vi "draw_quiver.vi"() -> ()   [LabVIEW 2016]
uses:
  <vilib>/Native 3D Graph/xcontrol/3DPC_SurfacePlot.xctl
  <vilib>/Native 3D Graph/classes/Line/Line.lvclass
panel:
  in  "XYZ Gain":dbl[](array[numeric])=[0.01, 0.01, 0.1]
  in  "XY Spacing":dbl=20.0 format="%#_13g"
  in  "Cols":i32=8
  in  "Rows":i32=8
  in  "Sensor Readings":dbl[][](array[numeric])=[[-533.0, -111.0, 239.0], [-402.0, 166.0, 184.0], [-184.0, 154.0, 29.0], [-106.0, 74.0, 11.0], [-532.0, -109.0, 246.0], [-398.0, 164.0, 175.0], [-205.0, 152.0, 32.0], [-119.0, 65.0, 9.0], [-529.0, -110.0, 242.0], [-408.0, 166.0, 184.0], [-198.0, 158.0, 27.0], [-108.0, 61.0, 6.0], [-539.0, -106.0, 240.0], [-407.0, 158.0, 183.0], [-191.0, 156.0, 28.0], [-113.0, 73.0, 15.0], [816.0, -260.0, 842.0], [539.0, 512.0, 512.0], [156.0, 425.0, 83.0], [13.0, 142.0, -72.0], [816.0, -262.0, 840.0], [528.0, 520.0, 512.0], [162.0, 425.0, 83.0], [13.0, 137.0, -84.0], [809.0, -260.0, 840.0], [538.0, 520.0, 504.0], [162.0, 432.0, 72.0], [13.0, 136.0, -84.0], [809.0, -260.0, 846.0], [538.0, 508.0, 512.0], [158.0, 435.0, 72.0], [19.0, 136.0, -79.0], [346.0, -168.0, 14.0], [287.0, -68.0, 19.0], [161.0, -34.0, 4.0], [70.0, -44.0, -7.0], [345.0, -191.0, 19.0], [279.0, -40.0, 8.0], [167.0, -16.0, 12.0], [72.0, -23.0, 2.0], [341.0, -190.0, 17.0], [285.0, -46.0, 9.0], [149.0, -15.0, 6.0], [54.0, -40.0, -2.0], [375.0, -201.0, 19.0], [282.0, -51.0, 10.0], [135.0, -37.0, 6.0], [81.0, -57.0, -12.0], [-80.0, -193.0, -48.0], [-73.0, -136.0, -12.0], [-5.0, -122.0, -31.0], [-19.0, -118.0, -17.0], [-118.0, -187.0, -48.0], [-73.0, -115.0, -22.0], [1.0, -113.0, -27.0], [-20.0, -111.0, -8.0], [-99.0, -184.0, -40.0], [-62.0, -145.0, -17.0], [0.0, -113.0, -37.0], [-7.0, -117.0, -15.0], [-126.0, -184.0, -50.0], [-72.0, -115.0, -14.0], [-4.0, -114.0, -25.0], [-29.0, -116.0, -14.0]]
  out "z vector":dbl[](array[numeric])=[0.0, 23.900000000000002, 0.0, 0.0, 18.400000000000002, 0.0, 0.0, 2.9000000000000004, 0.0, 0.0, 1.1, 0.0, 0.0, 24.6, 0.0, 0.0, 17.5, 0.0, 0.0, 3.2, 0.0, 0.0, 0.9, 0.0, 0.0, 24.200000000000003, 0.0, 0.0, 18.400000000000002, 0.0, 0.0, 2.7, 0.0, 0.0, 0.6000000000000001, 0.0, 0.0, 24.0, 0.0, 0.0, 18.3, 0.0, 0.0, 2.8000000000000003, 0.0, 0.0, 1.5, 0.0, 0.0, 84.2, 0.0, 0.0, 51.2, 0.0, 0.0, 8.3, 0.0, 0.0, -7.2, 0.0, 0.0, 84.0, 0.0, 0.0, 51.2, 0.0, 0.0, 8.3, 0.0, 0.0, -8.4, 0.0, 0.0, 84.0, 0.0, 0.0, 50.400000000000006, 0.0, 0.0, 7.2, 0.0, 0.0, -8.4, 0.0, 0.0, 84.60000000000001, 0.0, 0.0, 51.2, 0.0, 0.0, 7.2, 0.0, 0.0, -7.9, 0.0, 0.0, 1.4000000000000001, 0.0, 0.0, 1.9000000000000001, 0.0, 0.0, 0.4, 0.0, 0.0, -0.7000000000000001, 0.0, 0.0, 1.9000000000000001, 0.0, 0.0, 0.8, 0.0, 0.0, 1.2000000000000002, 0.0, 0.0, 0.2, 0.0, 0.0, 1.7000000000000002, 0.0, 0.0, 0.9, 0.0, 0.0, 0.6000000000000001, 0.0, 0.0, -0.2, 0.0, 0.0, 1.9000000000000001, 0.0, 0.0, 1.0, 0.0, 0.0, 0.6000000000000001, 0.0, 0.0, -1.2000000000000002, 0.0, 0.0, -4.800000000000001, 0.0, 0.0, -1.2000000000000002, 0.0, 0.0, -3.1, 0.0, 0.0, -1.7000000000000002, 0.0, 0.0, -4.800000000000001, 0.0, 0.0, -2.2, 0.0, 0.0, -2.7, 0.0, 0.0, -0.8, 0.0, 0.0, -4.0, 0.0, 0.0, -1.7000000000000002, 0.0, 0.0, -3.7, 0.0, 0.0, -1.5, 0.0, 0.0, -5.0, 0.0, 0.0, -1.4000000000000001, 0.0, 0.0, -2.5, 0.0, 0.0, -1.4000000000000001, 0.0]
  out "y vector":dbl[](array[numeric])=[0.0, -1.11, 0.0, 20.0, 21.66, 20.0, 40.0, 41.54, 40.0, 60.0, 60.74, 60.0, 80.0, 78.91, 80.0, 100.0, 101.64, 100.0, 120.0, 121.52, 120.0, 140.0, 140.65, 140.0, 0.0, -1.1, 0.0, 20.0, 21.66, 20.0, 40.0, 41.58, 40.0, 60.0, 60.61, 60.0, 80.0, 78.94, 80.0, 100.0, 101.58, 100.0, 120.0, 121.56, 120.0, 140.0, 140.73, 140.0, 0.0, -2.6, 0.0, 20.0, 25.12, 20.0, 40.0, 44.25, 40.0, 60.0, 61.42, 60.0, 80.0, 77.38, 80.0, 100.0, 105.2, 100.0, 120.0, 124.25, 120.0, 140.0, 141.37, 140.0, 0.0, -2.6, 0.0, 20.0, 25.2, 20.0, 40.0, 44.32, 40.0, 60.0, 61.36, 60.0, 80.0, 77.4, 80.0, 100.0, 105.08, 100.0, 120.0, 124.35, 120.0, 140.0, 141.36, 140.0, 0.0, -1.68, 0.0, 20.0, 19.32, 20.0, 40.0, 39.66, 40.0, 60.0, 59.56, 60.0, 80.0, 78.09, 80.0, 100.0, 99.6, 100.0, 120.0, 119.84, 120.0, 140.0, 139.77, 140.0, 0.0, -1.9000000000000001, 0.0, 20.0, 19.54, 20.0, 40.0, 39.85, 40.0, 60.0, 59.6, 60.0, 80.0, 77.99, 80.0, 100.0, 99.49, 100.0, 120.0, 119.63, 120.0, 140.0, 139.43, 140.0, 0.0, -1.93, 0.0, 20.0, 18.64, 20.0, 40.0, 38.78, 40.0, 60.0, 58.82, 60.0, 80.0, 78.13, 80.0, 100.0, 98.85, 100.0, 120.0, 118.87, 120.0, 140.0, 138.89, 140.0, 0.0, -1.84, 0.0, 20.0, 18.55, 20.0, 40.0, 38.87, 40.0, 60.0, 58.83, 60.0, 80.0, 78.16, 80.0, 100.0, 98.85, 100.0, 120.0, 118.86, 120.0, 140.0, 138.84, 140.0]
  out "x vector":dbl[](array[numeric])=[0.0, -5.33, 0.0, 0.0, -4.0200000000000005, 0.0, 0.0, -1.84, 0.0, 0.0, -1.06, 0.0, 0.0, -5.32, 0.0, 0.0, -3.98, 0.0, 0.0, -2.05, 0.0, 0.0, -1.19, 0.0, 20.0, 14.71, 20.0, 20.0, 15.92, 20.0, 20.0, 18.02, 20.0, 20.0, 18.92, 20.0, 20.0, 14.61, 20.0, 20.0, 15.93, 20.0, 20.0, 18.09, 20.0, 20.0, 18.87, 20.0, 40.0, 48.16, 40.0, 40.0, 45.39, 40.0, 40.0, 41.56, 40.0, 40.0, 40.13, 40.0, 40.0, 48.16, 40.0, 40.0, 45.28, 40.0, 40.0, 41.62, 40.0, 40.0, 40.13, 40.0, 60.0, 68.09, 60.0, 60.0, 65.38, 60.0, 60.0, 61.62, 60.0, 60.0, 60.13, 60.0, 60.0, 68.09, 60.0, 60.0, 65.38, 60.0, 60.0, 61.58, 60.0, 60.0, 60.19, 60.0, 80.0, 83.46, 80.0, 80.0, 82.87, 80.0, 80.0, 81.61, 80.0, 80.0, 80.7, 80.0, 80.0, 83.45, 80.0, 80.0, 82.79, 80.0, 80.0, 81.67, 80.0, 80.0, 80.72, 80.0, 100.0, 103.41, 100.0, 100.0, 102.85, 100.0, 100.0, 101.49, 100.0, 100.0, 100.54, 100.0, 100.0, 103.75, 100.0, 100.0, 102.82, 100.0, 100.0, 101.35, 100.0, 100.0, 100.81, 100.0, 120.0, 119.2, 120.0, 120.0, 119.27, 120.0, 120.0, 119.95, 120.0, 120.0, 119.81, 120.0, 120.0, 118.82, 120.0, 120.0, 119.27, 120.0, 120.0, 120.01, 120.0, 120.0, 119.8, 120.0, 140.0, 139.01, 140.0, 140.0, 139.38, 140.0, 140.0, 140.0, 140.0, 140.0, 139.93, 140.0, 140.0, 138.74, 140.0, 140.0, 139.28, 140.0, 140.0, 139.96, 140.0, 140.0, 139.71, 140.0]
  out "3D Graph":refnum<class "Base Datatype.lvclass">[](xcontrol)
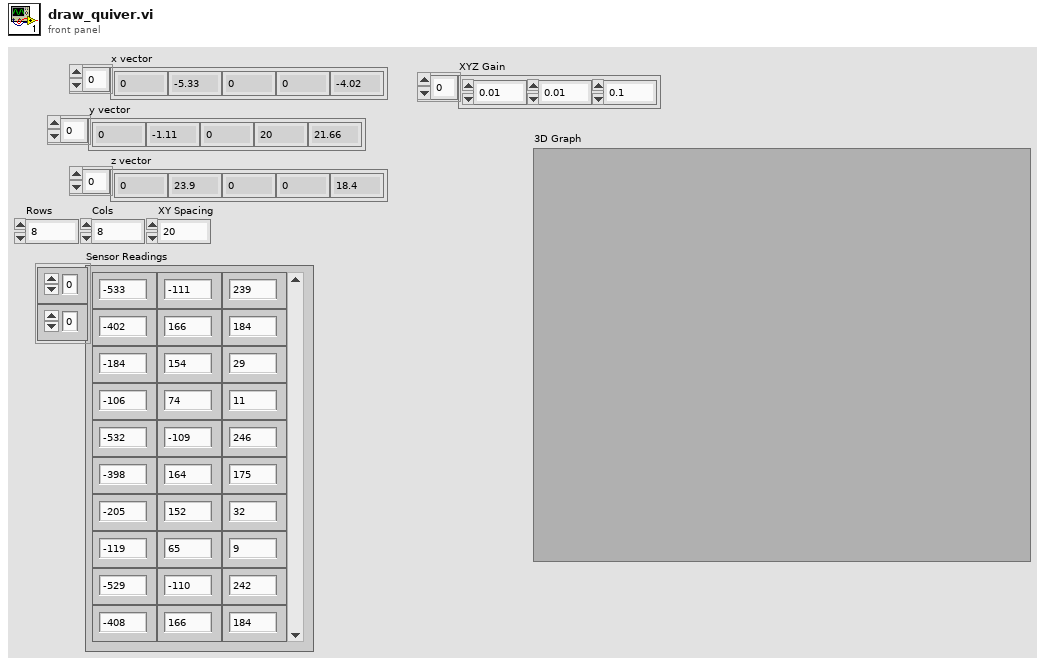
[diagram p1: front panel]
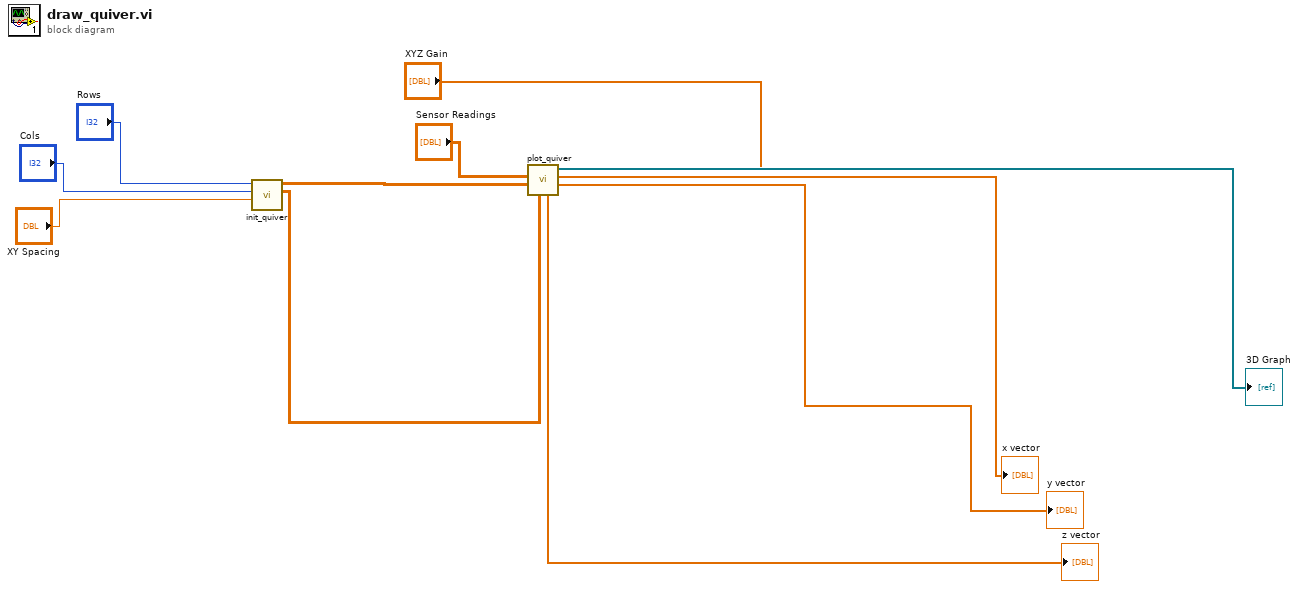
[diagram p0: block diagram]
diagram:
  n1 = call "init_quiver.vi"("XY Spacing"="XY Spacing", "Cols"="Cols", "Rows"="Rows") -> ("Quiver Data Prealloc"=w4:dbl[][], "Quiver Grid"=w8:dbl[][])  [unwired: 7 in]
  n2 = call "plot_quiver.vi"("Quiver Data Prealloc"=w4, "Quiver Grid"=w8, "Sensor Readings"="Sensor Readings", "XYZ Gain"="XYZ Gain") -> ("y vector"=→"y vector":dbl[], "x vector"=→"x vector":dbl[], "plots out"=→"3D Graph":refnum<class "Base Datatype.lvclass">[], "z vector"=→"z vector":dbl[])  [unwired: 4 in]
